vi "(SubVI) Find All Local Maximun_YCC.vi"(0 "Data Rate (Hz)":dbl, 1 "threshold y":dbl, 2 "Signal":dbl[](array[numeric]), 3 "Initial guess locations":i32[](array[numeric])) -> (6 "Total Peak location (index)":i32[](array[numeric]), 7 "Intervals Between Peaks":i32[](array[numeric]))   [LabVIEW 2014]
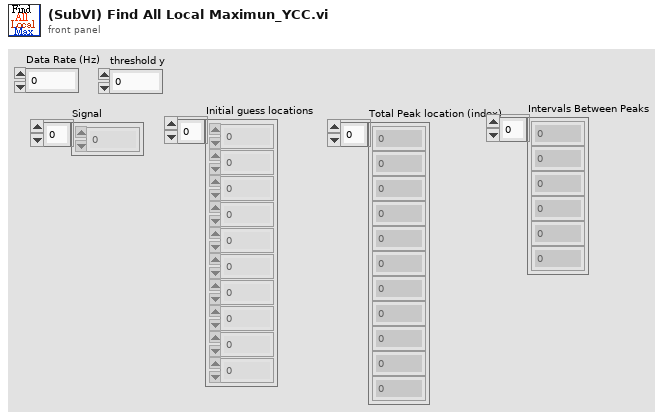
[diagram p1: front panel]
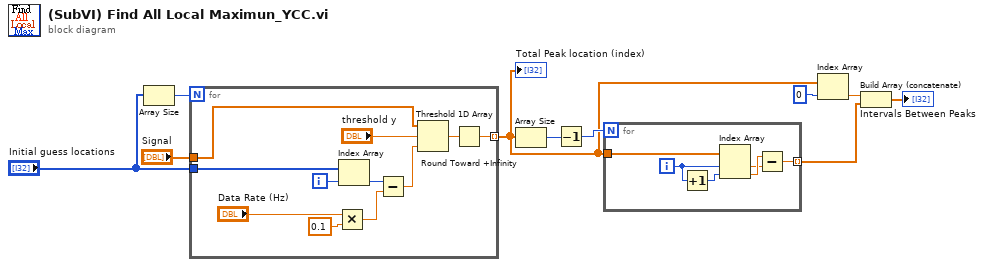
[diagram p0: block diagram]
diagram:
  n1 = Array Size(array="Initial guess locations") -> (size(s)=w9:i32)
  n2 = for {
    N: w9 -> [_]
    tunnel: [w18] -> w3 mode=indexing
    tunnel: "Signal" -> [w20]
    tunnel: "Initial guess locations" -> [w11]
    i -> [w17]
    n3 = Multiply(x="Data Rate (Hz)", y=0.1) -> (x*y=w13:dbl)
    n4 = Index Array(array=w11, index=w17) -> (element=w14:i32)
    n5 = Subtract(x=w14, y=w13) -> (x-y=w12:dbl)
    n6 = Threshold 1D Array(1:w12, 2:"threshold y", 3:w20) -> (0:w19:dbl)
    n7 = Round Toward +Infinity(x=w19) -> (ceil(x): smallest int >= x=w18:dbl)
  }
  "Total Peak location (index)" <- w3
  n8 = Array Size(array=w3) -> (size(s)=w7:i32)
  n9 = Decrement(x=w7) -> (x-1=w6:i32)
  n10 = for {
    N: w6 -> [_]
    tunnel: w3 -> [w27]
    tunnel: [w22] -> w5 mode=indexing
    i -> [w26]
    n11 = Increment(x=w26) -> (x+1=w25:i32)
    n12 = Index Array(array=w27, index #1=w26, index #2=w25) -> (element #1=w23:dbl, element #2=w24:dbl)
    n13 = Subtract(x=w24, y=w23) -> (x-y=w22:dbl)
  }
  n14 = Index Array(array=w3, index=0) -> (element=w2:dbl)
  n15 = Build Array (concatenate)(w2, w5) -> (→"Intervals Between Peaks":dbl[])
